vi "AutoMode.vi"   [LabVIEW 2024]
uses:
  DataTypes/OperationTypeForFunctionalGlobalVariable.ctl
types:
  T1 = typedef "OperationTypeForFunctionalGlobalVariable.ctl" = enum16{"GET", "SET"}
  T2 = enum16{"TOWARDS_0_DEGREES", "TOWARDS_180_DEGREES"}
  T3 = typedef "ServoStatus.ctl" = cluster{"mode":string, "position":i16}
  T4 = typedef "AutoModeParameters.ctl" = cluster{"movementDirection":enum16{"TOWARDS_0_DEGREES", "TOWARDS_180_DEGREES"}, "frequency":dbl}
  T5 = typedef "WebServiceStatus.ctl" = cluster{"isWebServiceShuttingDown":bool}
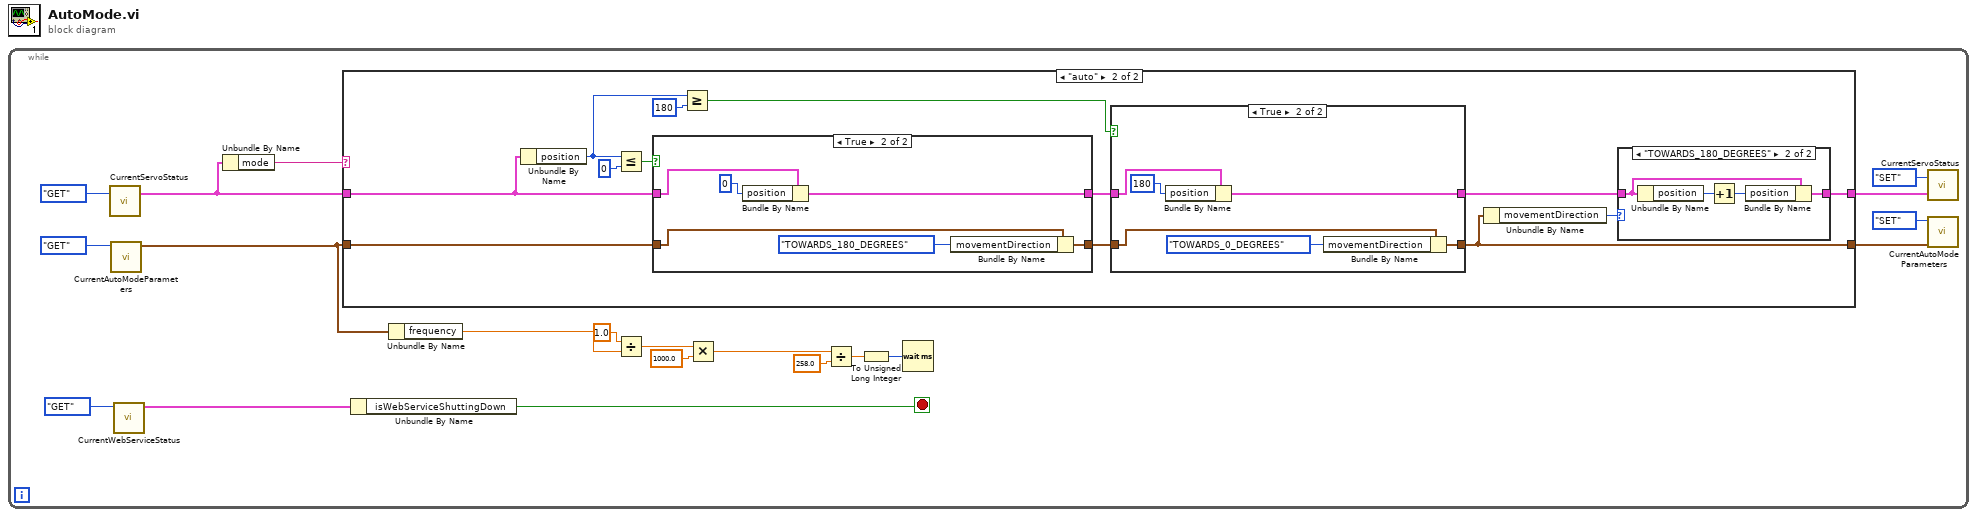
[diagram p0: block diagram]
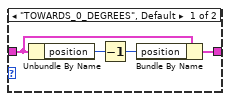
[diagram p5: hidden frame]
diagram:
  n1 = while {
    stop <- w1 stop-if-true
    n2 = call "CurrentServoStatus.vi"("Operation"=OperationTypeForFunctionalGlobalVariable."GET") -> ("Current Servo Status"=w14:T3)  [unwired: 2 in]
    n3 = call "CurrentAutoModeParameters.vi"("Operation"=OperationTypeForFunctionalGlobalVariable."GET") -> ("Current Auto Mode Parameters"=w16:T4)  [unwired: 10 in]
    n4 = call "CurrentWebServiceStatus.vi"("Operation"=OperationTypeForFunctionalGlobalVariable."GET") -> ("Current WebService Status"=w2:T5)  [unwired: 10 in]
    n5 = Unbundle By Name(w14) -> ("mode"=w15:string)
    n6 = case shown="\"auto\"" w15 {
      tunnel: w16 -> [w21 w25]
      tunnel: [w21 w23] -> w11
      tunnel: w14 -> [w22 w30]
      tunnel: [w22 w35] -> w12
      frame "manual", Default {
      }
      frame "auto" {
        n7 = Unbundle By Name(w30) -> ("position"=w32:i16)
        n8 = Less Or Equal?(x=w32, y=i16 0) -> (x <= y?=w31:bool)
        n9 = case shown="True" w31 {
          tunnel: w25 -> [w44 w50]
          tunnel: w30 -> [w45 w51]
          tunnel: [w45 w46] -> w29
          tunnel: [w44 w47] -> w27
          frame False {
          }
          frame True {
            n10 = Bundle By Name(cluster=w51, "position"=i16 0) -> (w46:T3)
            n11 = Bundle By Name(cluster=w50, "movementDirection"=T2."TOWARDS_180_DEGREES") -> (w47:T4)
          }
        }
        n12 = Greater Or Equal?(x=w32, y=i16 180) -> (x >= y?=w26:bool)
        n13 = case shown="True" w26 {
          tunnel: w27 -> [w36 w38]
          tunnel: w29 -> [w37 w39]
          tunnel: [w37 w41] -> w28
          tunnel: [w36 w40] -> w23
          frame False {
          }
          frame True {
            n14 = Bundle By Name(cluster=w39, "position"=i16 180) -> (w41:T3)
            n15 = Bundle By Name(cluster=w38, "movementDirection"=T2."TOWARDS_0_DEGREES") -> (w40:T4)
          }
        }
        n16 = Unbundle By Name(w23) -> ("movementDirection"=w24:T2)
        n17 = case shown="\"TOWARDS_180_DEGREES\"" w24 {
          tunnel: w28 -> [w52 w57]
          tunnel: [w53 w58] -> w35
          frame "TOWARDS_0_DEGREES", Default {
            n18 = Unbundle By Name(w52) -> ("position"=w55:i16)
            n19 = Decrement(x=w55) -> (x-1=w54:i16)
            n20 = Bundle By Name(cluster=w52, "position"=w54) -> (w53:T3)
          }
          frame "TOWARDS_180_DEGREES" {
            n21 = Unbundle By Name(w57) -> ("position"=w59:i16)
            n22 = Increment(x=w59) -> (x+1=w56:i16)
            n23 = Bundle By Name(cluster=w57, "position"=w56) -> (w58:T3)
          }
        }
      }
    }
    n24 = Unbundle By Name(w2) -> ("isWebServiceShuttingDown"=w1:bool)
    n25 = Unbundle By Name(w16) -> ("frequency"=w8:dbl)
    n26 = Divide(x=1.0, y=w8) -> (x/y=w7:dbl)
    n27 = Multiply(x=w7, y=1000.0) -> (x*y=w5:dbl)
    n28 = Divide(x=w5, y=258.0) -> (x/y=w4:dbl)
    n29 = To Unsigned Long Integer(number=w4) -> (unsigned 32bit integer=w19:u32)
    n30 = Wait (ms)(milliseconds to wait=w19) -> ()  [unwired: 1 out]
    n31 = call "CurrentServoStatus.vi"("New Servo Status"=w12, "Operation"=OperationTypeForFunctionalGlobalVariable."SET") -> ()  [unwired: 1 in, 1 out]
    n32 = call "CurrentAutoModeParameters.vi"("New Auto Mode Parameters"=w11, "Operation"=OperationTypeForFunctionalGlobalVariable."SET") -> ()  [unwired: 9 in, 1 out]
  }
